vi "Gyro Reset.vi"(11 "GyroDevRef":T1) -> ()   [LabVIEW 2014]
uses:
  <vilib>/Rock Robotics/WPI/Gyro/WPI_GyroDevRef.ctl
  <vilib>/Rock Robotics/SystemInterfaces/Typedef/FPGA_TypedefAnalogModule.ctl
  <vilib>/Rock Robotics/SystemInterfaces/AI/FPGA_AIChannel.ctl
  Robot Values.vi
  <vilib>/ptbypt/NI_PtbyPt.lvlib
panel:
  in  "Reset":bool
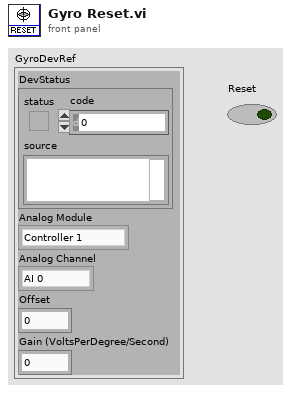
[diagram p1: front panel]
types:
  T1 = typedef "WPI_GyroDevRef.ctl" = cluster{"DevStatus":errorcluster, "Analog Module":T2, "Analog Channel":T3, "Offset":dbl, "Gain (VoltsPerDegree/Second)":dbl}
  T2 = typedef "FPGA_TypedefAnalogModule.ctl" = enum16{"Controller 1"}
  T3 = typedef "FPGA_AIChannel.ctl" = enum8{"AI 0", "AI 1", "AI 2", "AI 3", "AI MXP 0", "AI MXP 1", "AI MXP 2", "AI MXP 3", "Invalid"}
  T4 = cluster{"Lift Encoder Height Right (cm)":dbl, "Lift Encoder Height Left (cm)":dbl, "Right Prox":bool, "Left Prox":bool, "Gyro Angle":dbl, "Gyro anglar rate":dbl, "Gyro Reset":bool}
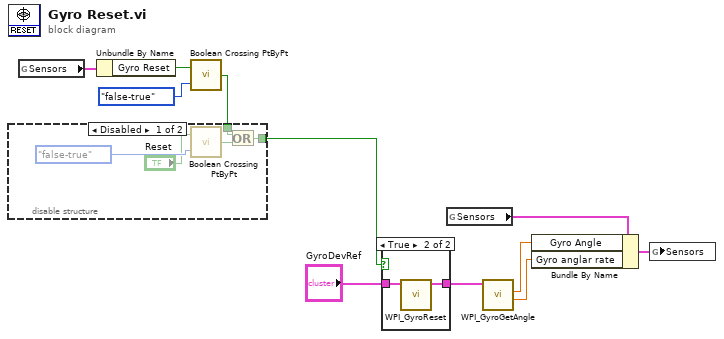
[diagram p0: block diagram]
diagram:
  n1 = global read "Robot Values.vi" "Sensors"() -> (w10:T4)
  n2 = Unbundle By Name(w10) -> ("Gyro Reset"=w3:bool)
  n3 = call <vilib>:"Boolean Crossing PtByPt.vi"("direction"=enum16{"either", "false-true", "true-false"}."false-true", "input"=w3) -> ("crossing"=w2:bool)  [unwired: 1 in]
  n4 = disable-structure shown="Disabled" {
    disable-tunnel: w2 -> [w13 w17]
    disable-tunnel: [w12 w17] -> w1
    frame Disabled {
      n5 = call <vilib>:"Boolean Crossing PtByPt.vi"("direction"=enum16{"either", "false-true", "true-false"}."false-true", "input"="Reset") -> ("crossing"=w14:bool)  [unwired: 1 in]
      n6 = Or(x=w13, y=w14) -> (x .or. y?=w12:bool)
    }
    frame Enabled {
    }
  }
  n7 = case shown="True" w1 {
    tunnel: "GyroDevRef" -> [w18 w20]
    tunnel: [w18 w19] -> w9
    frame False {
    }
    frame True {
      n8 = call <vilib>:"WPI_GyroReset.vi"("GyroDevRef"=w20) -> ("GyroDevRef"=w19:T1)  [unwired: 9 in, 1 out]
    }
  }
  n9 = global read "Robot Values.vi" "Sensors"() -> (w5:T4)
  n10 = call <vilib>:"WPI_GyroGetAngle.vi"("GyroDevRef"=w9) -> ("Angular Rate"=w7:dbl, "Angle"=w6:dbl)  [unwired: 7 in, 2 out]
  n11 = Bundle By Name(cluster=w5, "Gyro Angle"=w6, "Gyro anglar rate"=w7) -> (w4:T4)
  n12 = global write "Robot Values.vi" "Sensors"(w4) -> ()
